vi "Graph - Histogram.vi"() -> ()   [LabVIEW 2012]
doc: "Sample numeric display item."
uses:
  <vilib>/NI Veristand/Display Template Support/Display Template Support.llb/cluster_Screen Item Settings.ctl
  <vilib>/NI Veristand/Display Template Support/Display Template Support.llb/cluster_Graph Scale Settings.ctl
  <vilib>/NI Veristand/Display Template Support/Display Template Support.llb/cluster_Graph Plot Settings.ctl
  NationalInstruments.VeriStand.SystemStorage
  <vilib>/NI Veristand/Display Template Support/Display Template Support.llb/enum_Display Template Handler Minimal To Widget Msg.ctl
  <vilib>/NI Veristand/Display Template Support/Display Template Support.llb/enum_Display Template Handler Minimal To Workspace.ctl
  Workspace User Data.ctl
  <vilib>/NI Veristand/Display Template Support/Display Template Support.llb/sub_Display Template Handler Custom.vi
  <vilib>/NI Veristand/Execution/Workspace/NI VeriStand - Get Multiple Channel Values.vi
  <vilib>/NI Veristand/Execution/Workspace/NI_VS Workspace ExecutionAPI.lvlib
panel:
  out "Histogram Graph":cluster{"Array":dbl[], dbl[]}(graph)
  out "# Elements Out of Range":dbl
  in  "Gateway IP Address":string
  in  "NIVS.System Definition Root":refnum<k24>
  in  "Item.Data":T1
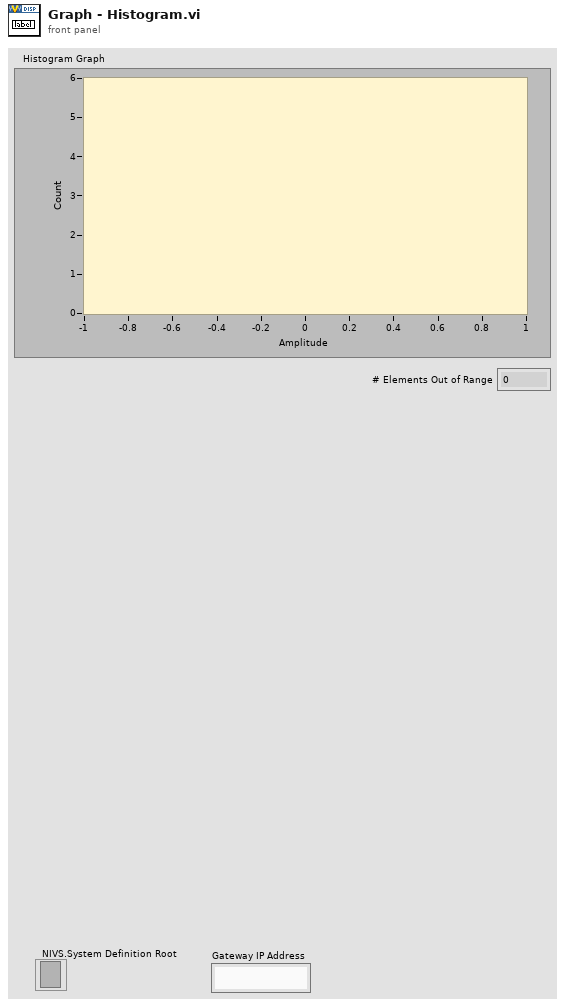
[diagram p1: front panel]
types:
  T1 = typedef "cluster_Screen Item Settings.ctl" = cluster{"Template VI":string, "Position X":i32, "Position Y":i32, "Custom":string, "Show Title Bar":bool, "ID":i32, "Always On Top":bool, "Allow Resize":bool, "Allow Minimize":bool, "Allow Close":bool, "Size to Screen":bool, "Screen.ID":i32, "State":enum16{"Normal", "New"}, "Title":string, "Window Bounds":cluster{"[0]":i16, "[1]":i16, "[2]":i16, "[3]":i16}, "Channel Ref":u64, "Unit":string, "Default Units?":bool, "Flash Limit?":bool, "Color 1":u32, "Color 2":u32, "Color 3":u32, "Color 4":u32, "Bck Color":u32, "Fore Color":u32, "Limit 1":dbl, "Limit 2":dbl, "Limit 3":dbl, "Limit 4":dbl, "Limit Mode 1":i32, "Limit Mode 2":i32, "Limit Mode 3":i32, "Limit Mode 4":i32, "Scale Precision":i32, "Scale Min":dbl, "Scale Max":dbl, "Format":i32, "Precision":i32, "Background Type":i32, "IDs":i32[], "Units":string[], "Labels":string[], "Scale Factor":dbl, "Scale Offset":dbl, "YScale Index":u32[], "XScale":T2, "YScales":T2[], "Plots":T3[], "Update Period":dbl, "History Length":dbl, "My.Ref":refnum<vi>, "Is Control?":bool, "Channel Paths":string[], "Custom Data":variant}
  T2 = typedef "cluster_Graph Scale Settings.ctl" = cluster{"Format":u8, "Precision":u8, "Fit":u8, "Label":string, "Use Default Label":bool, "Label Visible":bool, "Min":dbl, "Max":dbl}
  T3 = typedef "cluster_Graph Plot Settings.ctl" = cluster{"Bar Style":u8, "Fill To":i16, "Fill/PtColor":u32, "Line Style":u8, "Line Width":u8, "Color":u32, "Interp":u8, "Point Style":u8}
  T4 = typedef "enum_Display Template Handler Minimal To Workspace.ctl" = cluster{"Operation":enum16{"SetCustomData", "DeleteItem"}, "Data":variant}
  T5 = typedef "enum_Display Template Handler Minimal To Widget Msg.ctl" = enum16{"Stop", "LaunchConfigDialog"}
  T6 = typedef "Workspace User Data.ctl" = cluster{"Selected Item":string}
  T7 = typedef "NI_VS Workspace ExecutionAPI.lvlib/WorkspaceAPI.ctl" = refnum<k24>
  T8 = cluster{"Bin Counts":i32[], "Upper Bounds":dbl[], "Lower Bounds":dbl[]}
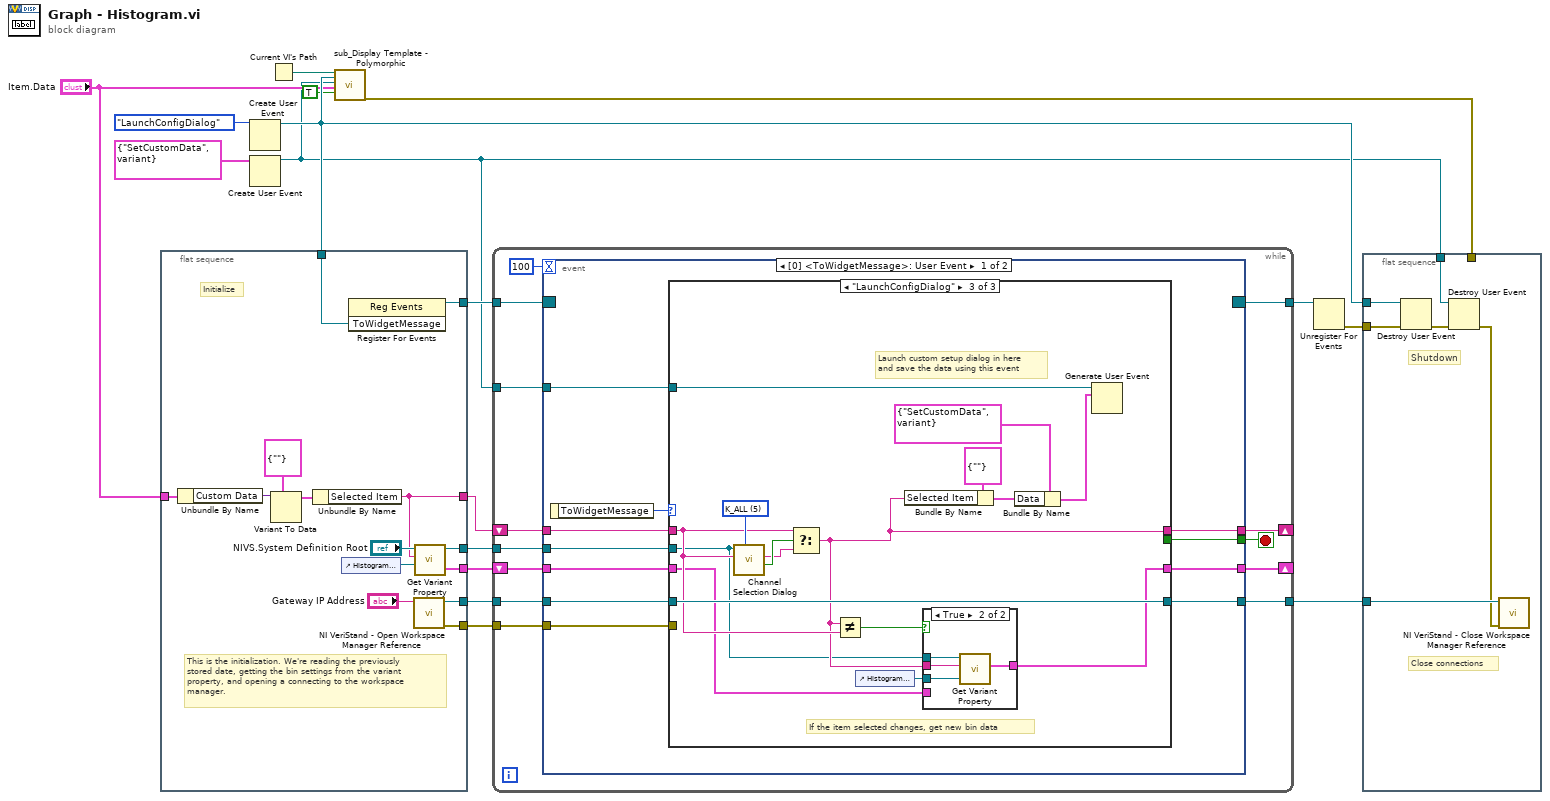
[diagram p0: block diagram]
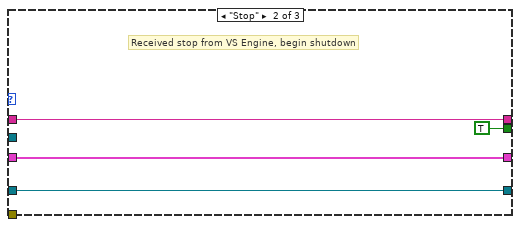
[diagram p3: hidden frame]
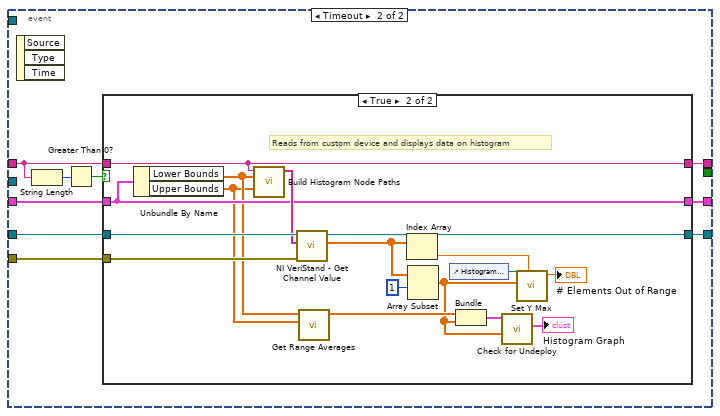
[diagram p5: hidden frame]
diagram:
  n1 = flat-sequence {
    tunnel: [w31] -> w15
    tunnel: w12 -> [w30]
    tunnel: "Item.Data" -> [w29]
    tunnel: [w21] -> w6
    tunnel: [w19] -> w5
    tunnel: [w25] -> w4
    tunnel: [w23] -> w3
    tunnel: [w20] -> w2
    frame #0 {
      # "This is the initialization. We're reading the previously\nstored date, getting the bin settings from the variant\nproperty, and opening a connecting to the workspace\nmanager."
      # "Initialize"
      n2 = Unbundle By Name(w29) -> ("Custom Data"=w28:variant)
      n3 = Variant To Data(type=T6 {"Selected Item"=""}, Variant=w28) -> (data=w26:T6)  [unwired: 1 in, 1 out]
      n4 = Unbundle By Name(w26) -> ("Selected Item"=w19:string)
      n5 = control-ref of="Histogram Graph"() -> (w18:refnum<vi>)
      n6 = register-events(w30) -> (reference out=w31:refnum<event-registration>)  [unwired: 2 in, 1 out]
      n7 = call <vilib>:"NI VeriStand - Open Workspace Manager Reference.vi"("Gateway IP Address (\"\": localhost)"="Gateway IP Address") -> ("error out"=w23:errorcluster, "WorkspaceManager"=w25:T7)  [unwired: 9 in]
      n8 = call "Get Variant Property.vi"("Histogram Graph Reference"=w18, "Selected Item"=w19, ".NET Refnum in"="NIVS.System Definition Root") -> ("Cluster"=w20:T8, ".NET Refnum out"=w21:refnum<k24>)  [unwired: 6 in, 1 out]
    }
  }
  n9 = Create User Event(user event datatype=enum_Display_Template_Handler_Minimal_To_Widget_Msg."LaunchConfigDialog" ("ToWidgetMessage")) -> (user event=w12:refnum<user-event>)  [unwired: 1 in, 1 out]
  n10 = Create User Event(user event datatype=T4 {"Operation"=enum."SetCustomData", "Data"=variant} ("Data")) -> (user event=w8:refnum<user-event>)  [unwired: 1 in, 1 out]
  n11 = Current VI's Path() -> (path=w10:path)
  n12 = call-poly <vilib>:"sub_Display Template - Polymorphic.vi"("Parent.Path"=w10, "ToWidgetEvent"=w12, "ToWorkspace"=w8, "Item.Data"="Item.Data", "Resizable"=TRUE) -> ("error out"=w17:errorcluster)  [unwired: 1 in, 13 out]
  n13 = while {
    tunnel: w15 -> [w44]
    tunnel: [w42] -> w14
    tunnel: w8 -> [w41]
    tunnel: w6 -> [w40]
    shift-right: [w38] -> _
    shift-left: w5 -> [w39]
    tunnel: w4 -> [w36]
    tunnel: w3 -> [w35]
    shift-right: [w33] -> _
    shift-left: w2 -> [w34]
    tunnel: [w32] -> w1
    stop <- w43 stop-if-true
    n14 = event shown="[0] <ToWidgetMessage>: User Event" {
      selector: w44 -> [_ _]
      dyn-events: [_ _] -> w42
      timeout: 100 -> [_ _]
      tunnel: [w54 _] -> w43
      tunnel: w41 -> [w53 _]
      tunnel: w40 -> [w52 _]
      tunnel: w39 -> [w51 w88]
      tunnel: [w50 w87] -> w38
      tunnel: w36 -> [w49 w90]
      tunnel: w35 -> [w48 w89]
      tunnel: w34 -> [w46 w86]
      tunnel: [w45 w85] -> w33
      tunnel: [w47 w84] -> w32
      event User Event {
        n15 = event-data() -> ("ToWidgetMessage"=w55:T5)  [unwired: 1 out]
        n16 = case shown="\"LaunchConfigDialog\"" w55 {
          tunnel: [_ TRUE _] -> w54
          tunnel: w53 -> [_ _ w78]
          tunnel: w52 -> [_ _ w65]
          tunnel: w51 -> [w58 w61 w69]
          tunnel: [w58 w61 w66] -> w50
          tunnel: w49 -> [w57 w60 w70]
          tunnel: w48 -> [_ _ _]
          tunnel: [w57 w60 w70] -> w47
          tunnel: w46 -> [w56 w59 w68]
          tunnel: [w56 w59 w64] -> w45
          frame Default {
            # "Do Nothing"
          }
          frame "Stop" {
            # "Received stop from VS Engine, begin shutdown"
          }
          frame "LaunchConfigDialog" {
            w71 = u8 5 items=["K_CHAN_R", "K_CHAN_W", "K_CHAN_RW", "K_CHAN_VOLT", "K_CHAN_FAULT", "K_ALL", "K_CUSTOM", "K_CHAN_R_VIS", "K_CHAN_W_VIS", "K_CHAN_RW_VIS", "K_CHAN_VOLT_VIS", "K_CHAN_FAULT_VIS"] ("DisplayFilter")
            # "If the item selected changes, get new bin data"
            # "Launch custom setup dialog in here\nand save the data using this event"
            n17 = call "Channel Selection Dialog.vi"("DisplayFilter"=w71, "Current selection"=w69, "NIVS.System Definition Root"=w65) -> ("Cancelled"=w73:bool, "New selection"=w72:string)  [unwired: 6 in, 1 out]
            n18 = Select(t=w69, s=w73, f=w72) -> (s? t:f=w66:string)
            n19 = Not Equal?(x=w66, y=w69) -> (x != y?=w67:bool)
            n20 = control-ref of="Histogram Graph"() -> (w63:refnum<vi>)
            n21 = Bundle By Name(cluster=T6 {"Selected Item"=""}, "Selected Item"=w66) -> (w74:T6)
            n22 = case shown="True" w67 {
              tunnel: w68 -> [w79 _]
              tunnel: w66 -> [_ w83]
              tunnel: w65 -> [_ w82]
              tunnel: [w79 w81] -> w64
              tunnel: w63 -> [_ w80]
              frame False {
              }
              frame True {
                n23 = call "Get Variant Property.vi"("Histogram Graph Reference"=w80, "Selected Item"=w83, ".NET Refnum in"=w82) -> ("Cluster"=w81:T8)  [unwired: 6 in, 2 out]
              }
            }
            n24 = Bundle By Name(cluster=T4 {"Operation"=enum."SetCustomData", "Data"=variant} ("event data"), "Data"=w74) -> (w76:T4)
            n25 = Generate User Event(user event=w78, event data cluster=w76) -> ()  [unwired: 1 in, 2 out]
          }
        }
      }
      event Timeout {
        n26 = event-data() -> ()  [unwired: 4 out]
        n27 = String Length(string=w88) -> (length=w92:i32)
        n28 = Greater Than 0?(x=w92) -> (x > 0?=w91:bool)
        n29 = case shown="True" w91 {
          tunnel: w90 -> [w93 w111]
          tunnel: w89 -> [_ w109]
          tunnel: w88 -> [w95 w112]
          tunnel: [w95 w112] -> w87
          tunnel: w86 -> [w94 w104]
          tunnel: [w94 w104] -> w85
          tunnel: [w93 w105] -> w84
          frame False {
            # "No Histogram Custom Device has been selected. Do Nothing"
          }
          frame True {
            # "Reads from custom device and displays data on histogram"
            n30 = Unbundle By Name(w104) -> ("Lower Bounds"=w103:dbl[], "Upper Bounds"=w102:dbl[])
            n31 = call "Build Histogram Node Paths.vi"("Upper Bounds"=w102, "Lower Bounds"=w103, "Selected Item"=w112) -> ("Node Paths"=w110:string[])  [unwired: 8 in]
            n32 = call-poly <vilib>:"NI VeriStand - Get Channel Value.vi"("error in (no error)"=w109, "Channels"=w110, "WorkspaceManager in"=w111) -> ("Values"=w107:dbl[], "WorkspaceManager out"=w105:T7)  [unwired: 6 in, 1 out]
            n33 = call "Get Range Averages.vi"("Upper Bounds"=w102, "Lower Bounds"=w103) -> ("Array"=w108:dbl[])  [unwired: 9 in]
            n34 = Index Array(array=w107) -> (element=w97:dbl)  [unwired: 1 in]
            n35 = Array Subset(array=w107, index=1) -> (w98:dbl[])  [unwired: 1 in]
            n36 = control-ref of="Histogram Graph"() -> (w101:refnum<vi>)
            n37 = Bundle("Array"=w108, w98) -> (w99:cluster{"Array":dbl[], dbl[]})  [unwired: 1 in]
            n38 = call "Check for Undeploy.vi"("Histogram Data"=w98, "Histogram In"=w99) -> ("Histogram Out"=→"Histogram Graph":cluster{"Array":dbl[], dbl[]})  [unwired: 9 in]
            n39 = call "Set Y Max.vi"("# Elem"=w97, "Array"=w98, "XYGraph in"=w101) -> ("# Elem Out"=→"# Elements Out of Range":dbl)  [unwired: 8 in]
          }
        }
      }
    }
  }
  n40 = Unregister For Events(event registration refnum=w14) -> (error out=w13:errorcluster)  [unwired: 1 in]
  n41 = flat-sequence {
    tunnel: w17 -> [_]
    tunnel: w13 -> [w117]
    tunnel: w12 -> [w118]
    tunnel: w8 -> [w115]
    tunnel: w1 -> [w114]
    frame #0 {
      # "Close connections"
      # "Shutdown"
      n42 = Destroy User Event(user event=w118, error in=w117) -> (error out=w116:errorcluster)
      n43 = Destroy User Event(user event=w115, error in=w116) -> (error out=w113:errorcluster)
      n44 = call <vilib>:"NI VeriStand - Close Workspace Manager Reference.vi"("error in (no error)"=w113, "WorkspaceManager"=w114) -> ()  [unwired: 9 in, 1 out]
    }
  }
